vi "CURVA S.vi"(0 "VISA Refnum in":refnum<visa-resource-name>, 1 "1st curve parameters":T1, 2 "2nd curve parameters":T1, 3 "error in (no error)":errorcluster, 4 "Grupo":u32) -> (5 "VISA Refnum out":refnum<visa-resource-name>, 6 "error out":errorcluster)   [LabVIEW 2014]
uses:
  <userlib>/Newport ESP301/Newport ESP301.lvlib
panel:
  out "y":i32
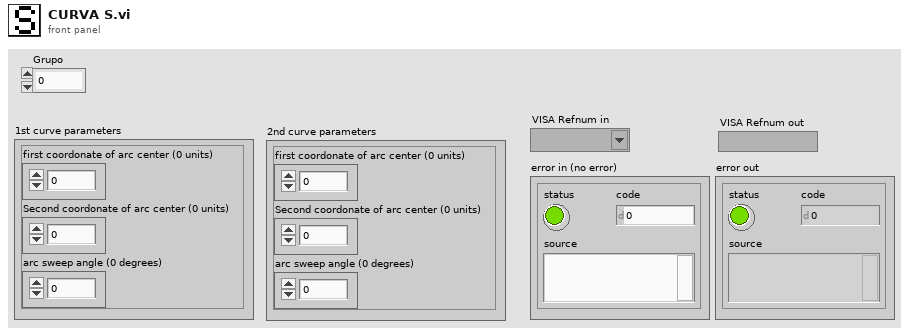
[diagram p1: front panel]
types:
  T1 = cluster{"first coordonate of arc center (0 units)":dbl, "Second coordonate of arc center (0 units)":dbl, "arc sweep angle (0 degrees)":dbl}
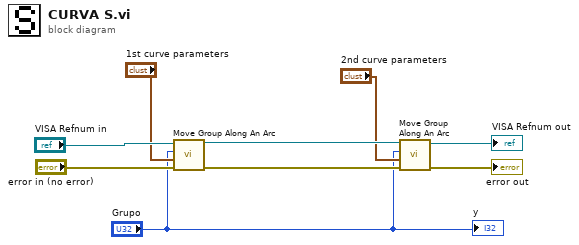
[diagram p0: block diagram]
diagram:
  n1 = call <userlib>:"Move Group Along An Arc.vi"("error in (no error)"="error in (no error)", "Arc  Parameters"="1st curve parameters", "Group Number (1)"="Grupo", "VISA resource name"="VISA Refnum in") -> ("error out"=w9:errorcluster, "VISA resource name out"=w8:refnum<visa-resource-name>)  [unwired: 2 in]
  n2 = call <userlib>:"Move Group Along An Arc.vi"("error in (no error)"=w9, "Arc  Parameters"="2nd curve parameters", "Group Number (1)"="Grupo", "VISA resource name"=w8) -> ("error out"=→"error out":errorcluster, "VISA resource name out"=→"VISA Refnum out":refnum<visa-resource-name>)  [unwired: 2 in]
  "y" <- "Grupo"
